vi "Get Chnl by Name.vi"(0 "BME_DG_System in":refnum<class "BME_DG_System.lvclass">, 5 "Chnl Name":string, 11 "error in (no error)":errorcluster) -> (4 "BME_DG_System out":refnum<class "BME_DG_System.lvclass">, 6 "BME_DG_Chnl":refnum<class "BME_DG_Chnl.lvclass">, 8 "Owner DG":refnum<class "BME_DG_Base.lvclass">, 10 "found?":bool, 14 "Master DG":refnum<class "BME_DG_Base.lvclass">, 15 "error out":errorcluster)   [LabVIEW 2009, in "POLARIS BME DG.lvlib" / "BME_DG_System.lvclass"]
uses:
  BME_DG_System.lvclass
  BME_DG_Base/BME_DG_Base.lvclass
  BME_DG_Chnl/BME_DG_Chnl.lvclass
  BME_DG_System.lvclass/BME_DG_System.ctl
  POLARIS BME DG.lvlib
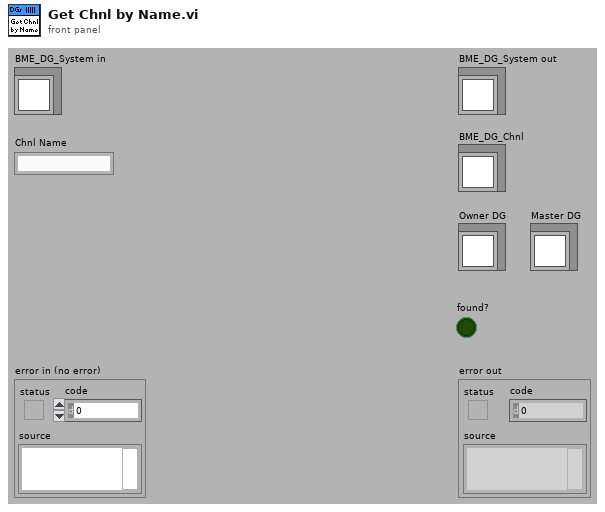
[diagram p1: front panel]
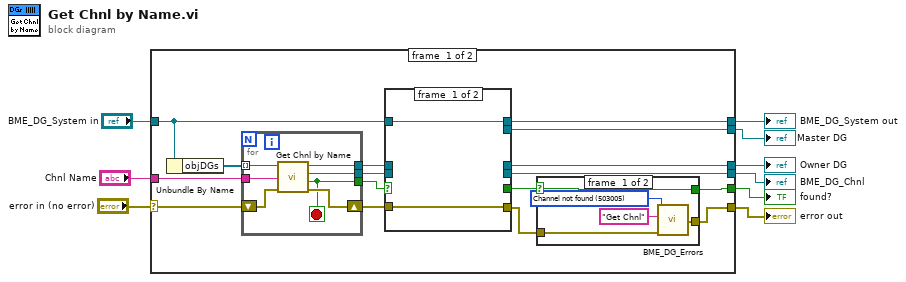
[diagram p0: block diagram]
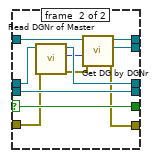
[diagram p3: hidden frame]
diagram:
  n1 = case shown="No Error" "error in (no error)" {
    selector: "error in (no error)" -> [w24 w54]
    tunnel: [w12 w54] -> w8
    tunnel: [w16 w53] -> w6
    tunnel: "BME_DG_System in" -> [w17 w53]
    tunnel: "Chnl Name" -> [w23 _]
    tunnel: [w21 _] -> w2
    tunnel: [w18 _] -> w3
    tunnel: [w10 _] -> w4
    tunnel: [w14 _] -> w1
    frame #0 {
      n2 = Unbundle By Name(w17) -> ("objDGs"=w25:refnum<class "BME_DG_Base.lvclass">[])
      n3 = for {
        tunnel: w25 -> [w52] mode=indexing
        shift-right: [w50] -> w15
        shift-left: w24 -> [w51]
        tunnel: [w49] -> w22
        tunnel: w23 -> [w48]
        tunnel: [w47] -> w20
        tunnel: [w46] -> w19
        stop <- w49 stop-if-true
        n4 = call-dynamic "Get Chnl by Name.vi"("error in (no error)"=w51, "Chnl Name"=w48, "BME_DG_Base in"=w52) -> ("error out"=w50:errorcluster, "found?"=w49:bool, "BME_DG_Chnl out"=w46:refnum<class "BME_DG_Chnl.lvclass">, "BME_DG_Base out"=w47:refnum<class "BME_DG_Base.lvclass">)  [unwired: 5 in]
      }
      n5 = case shown="True" w22 {
        selector: w22 -> [_ w44]
        tunnel: [_ w40] -> w21
        tunnel: w20 -> [_ w41]
        tunnel: [_ w45] -> w18
        tunnel: w19 -> [_ w45]
        tunnel: [_ w44] -> w11
        tunnel: w17 -> [w34 w43]
        tunnel: [w34 w42] -> w16
        tunnel: w15 -> [w33 w37]
        tunnel: [w33 w36] -> w13
        tunnel: [_ w35] -> w14
        frame #0 {
        }
        frame #1 {
          n6 = call-dynamic "Read DGNr of Master.vi"("error in (no error)"=w37, "BME_DG_Base in"=w41) -> ("error out"=w38:errorcluster, "DGNr of Master"=w39:i32, "BME_DG_Base out"=w40:refnum<class "BME_DG_Base.lvclass">)  [unwired: 7 in]
          n7 = call "Get DG by DGNr.vi"("error in (no error)"=w38, "DG Nr."=w39, "BME_DG_System in"=w43) -> ("error out"=w36:errorcluster, "BME_DG_Base.lvclass"=w35:refnum<class "BME_DG_Base.lvclass">, "BME_DG_System out"=w42:refnum<class "BME_DG_System.lvclass">)  [unwired: 5 in, 1 out]
        }
      }
      n8 = case shown="False" w11 {
        selector: w11 -> [w28 w31]
        tunnel: w13 -> [w30 w32]
        tunnel: [w29 w32] -> w12
        tunnel: [w28 w31] -> w10
        frame #0 {
          w26 = 503005 items=["Channel refers itself"=503001, "Deadloop"=503002, "Negative Delay"=503003, "Delay Card not found"=503004, "Channel not found"=503005] ("error")
          n9 = call "BME_DG_Errors.vi"("error in (no error)"=w30, "source"="Get Chnl", "error"=w26) -> ("error out"=w29:errorcluster)  [unwired: 8 in]
        }
        frame #1 {
        }
      }
    }
    frame #1 {
    }
  }
  "error out" <- w8
  "BME_DG_System out" <- w6
  "BME_DG_Chnl" <- w3
  "Owner DG" <- w2
  "found?" <- w4
  "Master DG" <- w1
